vi "Msg.Q.Enqueue.vi"(8 "error in (no error)":errorcluster, 9 "Data":variant, 10 "Message":string, 11 "Messaging in":refnum<class "Messaging.lvclass">) -> (0 "error out":errorcluster, 3 "Messaging out":refnum<class "Messaging.lvclass">)   [LabVIEW 2023, in "Messaging.lvclass"]
uses:
  Messaging.lvclass
  Messaging.lvclass/Messaging.ctl
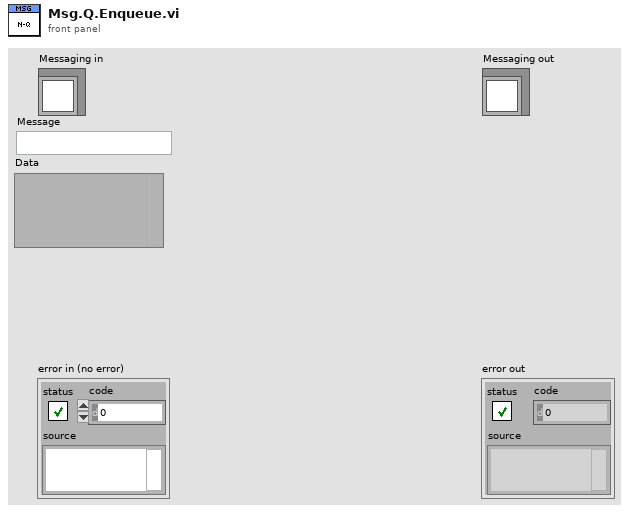
[diagram p1: front panel]
types:
  T1 = typedef "Msg.Q.Ref.ctl" = refnum<queue>
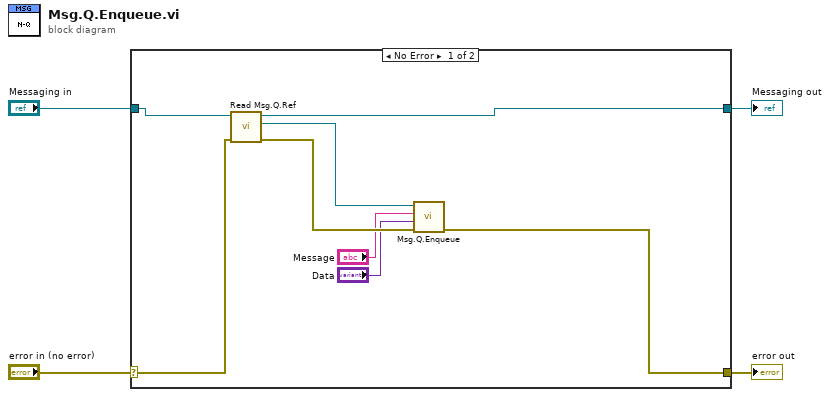
[diagram p0: block diagram]
diagram:
  n1 = case shown="No Error" "error in (no error)" {
    selector: "error in (no error)" -> [w9 w14]
    tunnel: [w7 w14] -> w3
    tunnel: [w10 w13] -> w1
    tunnel: "Messaging in" -> [w12 w13]
    frame No Error {
      n2 = call-dynamic "Read Msg.Q.Ref.vi"("error in (no error)"=w9, "Messaging in"=w12) -> ("error out"=w8:errorcluster, "Msg.Q.Ref"=w11:T1, "Messaging out"=w10:refnum<class "Messaging.lvclass">)  [unwired: 7 in]
      n3 = call "Msg.Q.Enqueue.vi"("Error (in)"=w8, "Data"="Data", "Message"="Message", "Msg.Q.Ref"=w11) -> ("Error (out)"=w7:errorcluster)  [unwired: 6 in, 1 out]
    }
    frame Error {
    }
  }
  "error out" <- w3
  "Messaging out" <- w1
